vi "System Setup.vi"(8 "error in (no error)":errorcluster, 11 "Set Oscillator":T1) -> (0 "error out":errorcluster)   [LabVIEW 2015]
uses:
  Oscillator.ctl
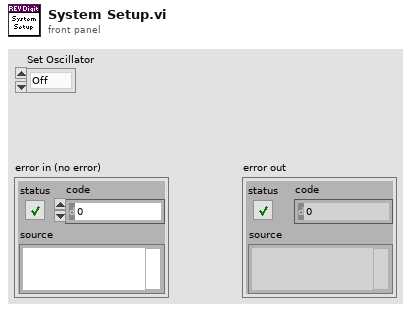
[diagram p1: front panel]
types:
  T1 = typedef "Oscillator.ctl" = enum16{"Off", "On"}
  T2 = typedef "WPI_I2CDevRef.ctl" = cluster{"DevStatus":errorcluster, "Device Address":u8, "Handle":i32, "I2C Bus":T3}
  T3 = typedef "i2c_bus.ctl" = enum16{"I2C On-Board", "I2C MXP", "Invalid"}
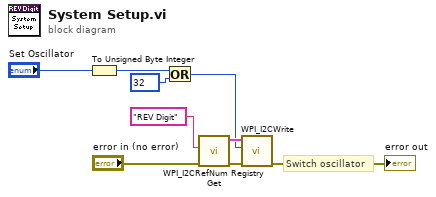
[diagram p0: block diagram]
diagram:
  # "Switch oscillator"
  n1 = To Unsigned Byte Integer(number="Set Oscillator") -> (unsigned 8bit integer=w5:u8)
  n2 = Or(x=w5, y=u8 32 ("I2CRegister")) -> (x .or. y?=w3:u8)
  n3 = call <vilib>:"WPI_I2CRefNum Registry Get.vi"("error in (no error)"="error in (no error)", "refnum name"="REV Digit") -> ("error out"=w9:errorcluster, "I2CDevRef"=w8:T2)  [unwired: 8 in]
  n4 = call <vilib>:"WPI_I2CWrite.vi"("error in (no error)"=w9, "I2CRegister"=w3, "I2CDevRef"=w8) -> ("error out"=→"error out":errorcluster)  [unwired: 7 in, 1 out]
